vi "SetSpeedQueue.vi"(0 "MotorNum队列":refnum<queue>, 5 "MotorSpeed队列":refnum<queue>, 7 "MotorNum元素":i32, 9 "MotorSpeed元素":i32, 11 "错误输入（无错误）":errorcluster) -> (4 "MotorNum队列输出":refnum<queue>, 6 "MotorSpeed队列输出":refnum<queue>, 15 "错误输出":errorcluster)   [LabVIEW 2011]
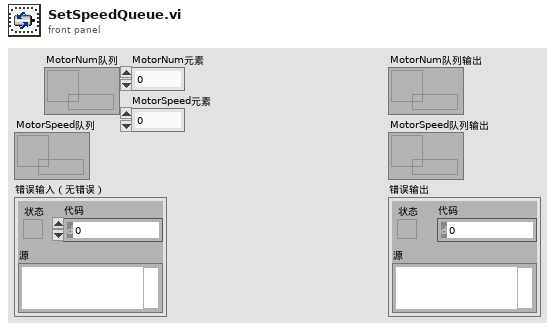
[diagram p1: front panel]
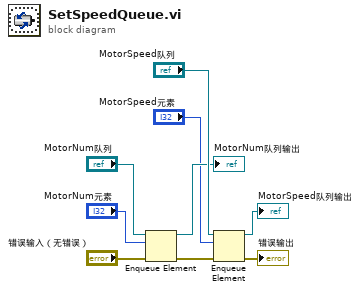
[diagram p0: block diagram]
diagram:
  n1 = Enqueue Element(queue="MotorNum队列", element="MotorNum元素", error in (no error)="错误输入（无错误）") -> (queue out=→"MotorNum队列输出":refnum<queue>, error out=w7:errorcluster)  [unwired: 1 in, 1 out]
  n2 = Enqueue Element(queue="MotorSpeed队列", element="MotorSpeed元素", error in (no error)=w7) -> (queue out=→"MotorSpeed队列输出":refnum<queue>, error out=→"错误输出":errorcluster)  [unwired: 1 in, 1 out]
